vi "read_write path.vi"(0 "laser rough cutting":path, 1 "making by hot":path, 2 "laser fine cutting":path, 3 "PDF":path, 4 "roll":path, 5 "EOL":path, 6 "type(read)":enum16{"read", "write"}(ring)) -> (14 "laser rough cutting":path, 15 "making by hot":path, 16 "laser fine cutting":path, 17 "PDF":path, 18 "roll":path, 19 "EOL":path)   [LabVIEW 2014]
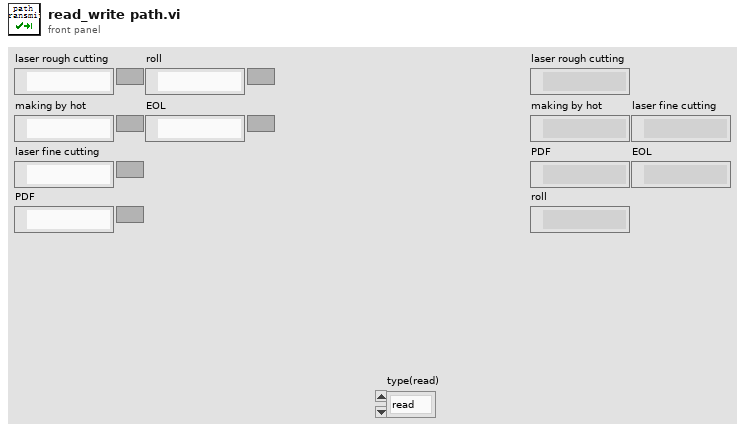
[diagram p1: front panel]
types:
  T1 = cluster{"laser rough cutting":path, "making by hot":path, "laser fine cutting":path, "PDF":path, "roll":path, "EOL":path}
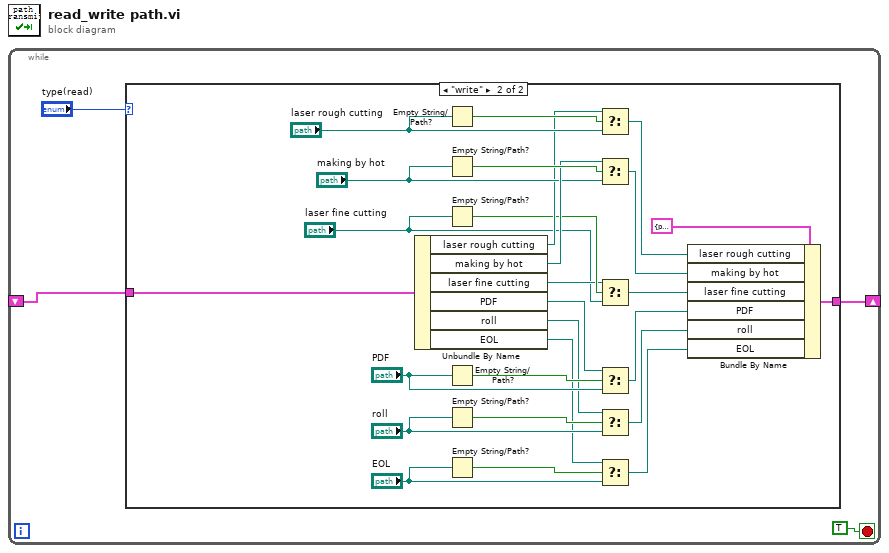
[diagram p0: block diagram]
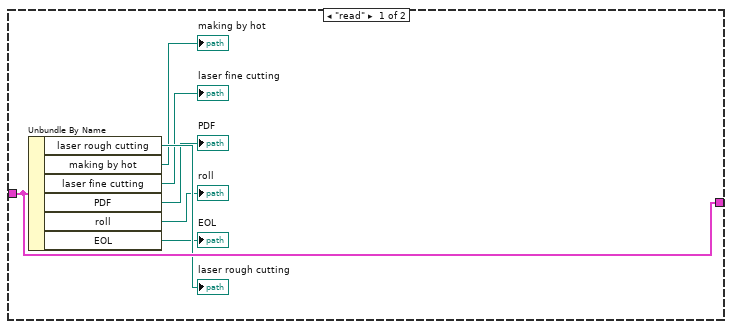
[diagram p2: hidden frame]
diagram:
  n1 = while {
    shift-right: [w3] -> _
    shift-left: _ -> [w2]
    stop <- TRUE stop-if-true
    n2 = case shown="\"write\"" "type(read)" {
      tunnel: [w11 w38] -> w3
      tunnel: w2 -> [w11 w36]
      frame "read" {
        n3 = Unbundle By Name(w11) -> ("laser rough cutting"=→"laser rough cutting":path, "making by hot"=→"making by hot":path, "laser fine cutting"=→"laser fine cutting":path, "PDF"=→"PDF":path, "roll"=→"roll":path, "EOL"=→"EOL":path)
      }
      frame "write" {
        n4 = Unbundle By Name(w36) -> ("laser rough cutting"=w28:path, "making by hot"=w31:path, "laser fine cutting"=w26:path, "PDF"=w22:path, "roll"=w18:path, "EOL"=w14:path)
        n5 = Empty String/Path?(string/path="laser rough cutting") -> (empty?=w35:bool)
        n6 = Empty String/Path?(string/path="making by hot") -> (empty?=w32:bool)
        n7 = Empty String/Path?(string/path="laser fine cutting") -> (empty?=w27:bool)
        n8 = Empty String/Path?(string/path="PDF") -> (empty?=w23:bool)
        n9 = Empty String/Path?(string/path="roll") -> (empty?=w19:bool)
        n10 = Empty String/Path?(string/path="EOL") -> (empty?=w15:bool)
        n11 = Select(t=w28, s=w35, f="laser rough cutting") -> (s? t:f=w33:path)
        n12 = Select(t=w31, s=w32, f="making by hot") -> (s? t:f=w29:path)
        n13 = Select(t=w26, s=w27, f="laser fine cutting") -> (s? t:f=w24:path)
        n14 = Select(t=w22, s=w23, f="PDF") -> (s? t:f=w20:path)
        n15 = Select(t=w18, s=w19, f="roll") -> (s? t:f=w16:path)
        n16 = Select(t=w14, s=w15, f="EOL") -> (s? t:f=w12:path)
        n17 = Bundle By Name(cluster=T1 {"laser rough cutting"=path "", "making by hot"=path "", "laser fine cutting"=path "", "PDF"=path "", "roll"=path "", "EOL"=path ""}, "laser rough cutting"=w33, "making by hot"=w29, "laser fine cutting"=w24, "PDF"=w20, "roll"=w16, "EOL"=w12) -> (w38:T1)
      }
    }
  }
